vi "Send Response.vi"(6 "overwrite on timeout (T)":bool, 8 "error in (no error)":errorcluster, 9 "timeout in ms (0)":i32, 10 "response data":u8[](array[numeric]), 11 "Interface in":refnum<class "Interface.lvclass">) -> (0 "error out":errorcluster, 1 "timed out?":bool, 3 "Interface out":refnum<class "Interface.lvclass">, 4 "# elements":u32)   [LabVIEW 2021, in "DSF Core.lvlib" / "Interface.lvclass"]
uses:
  Interface.lvclass
  Interface.lvclass/Interface.ctl
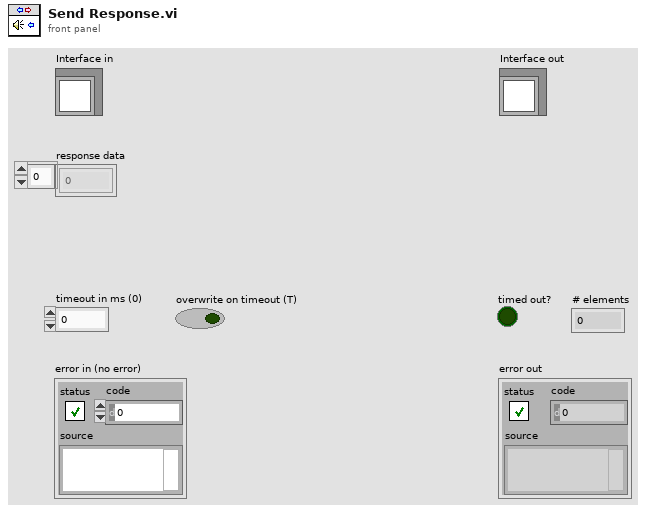
[diagram p1: front panel]
types:
  T1 = typedef "DSF Core.lvlib/Framework.lvclass/DSF FIFO Options.ctl" = cluster{"Infinite Timeouts":bool}
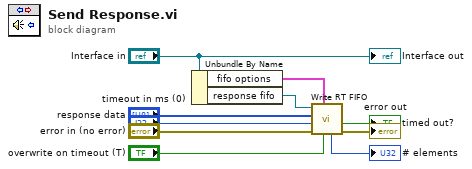
[diagram p0: block diagram]
diagram:
  n1 = Unbundle By Name("Interface in") -> ("fifo options"=w3:T1, "response fifo"=w4:refnum<k33>)
  n2 = call "Write RT FIFO.vi"("overwrite on timeout (T)"="overwrite on timeout (T)", "fifo options"=w3, "error in (no error)"="error in (no error)", "timeout in ms (0)"="timeout in ms (0)", "element"="response data", "rt fifo in"=w4) -> ("error out"=→"error out":errorcluster, "timed out?"=→"timed out?":bool, "# elements"=→"# elements":u32)  [unwired: 2 in, 1 out]
  "Interface out" <- "Interface in"
